vi "colourByStage.vi"(8 "error in (no error)":errorcluster, 11 "ScriptEditorV2 in":refnum<class "ScriptEditorV2.lvclass">) -> (0 "error out":errorcluster, 3 "ScriptEditorV2 out":refnum<class "ScriptEditorV2.lvclass">)   [LabVIEW 2009, in "Views.lvlib" / "ScriptEditor.lvlib" / "ScriptEditorV2.lvclass"]
uses:
  ScriptEditorV2.lvclass
  ScriptEditorV2.lvclass/ScriptEditorV2.ctl
  Tools/DatabaseHelpers/DbConnection/DeviceDataBase/deviceDataBase.lvclass
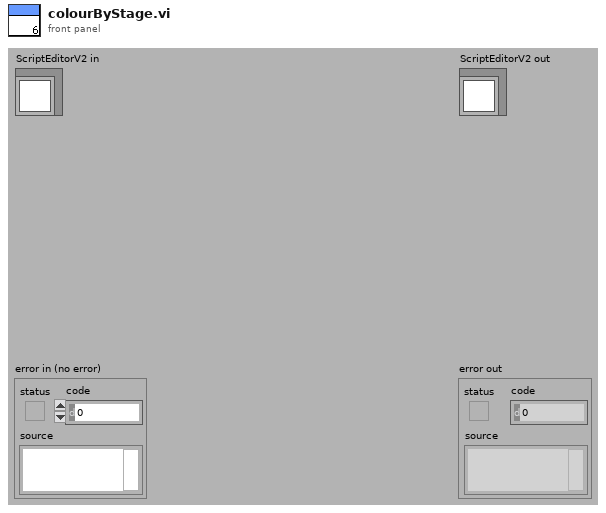
[diagram p1: front panel]
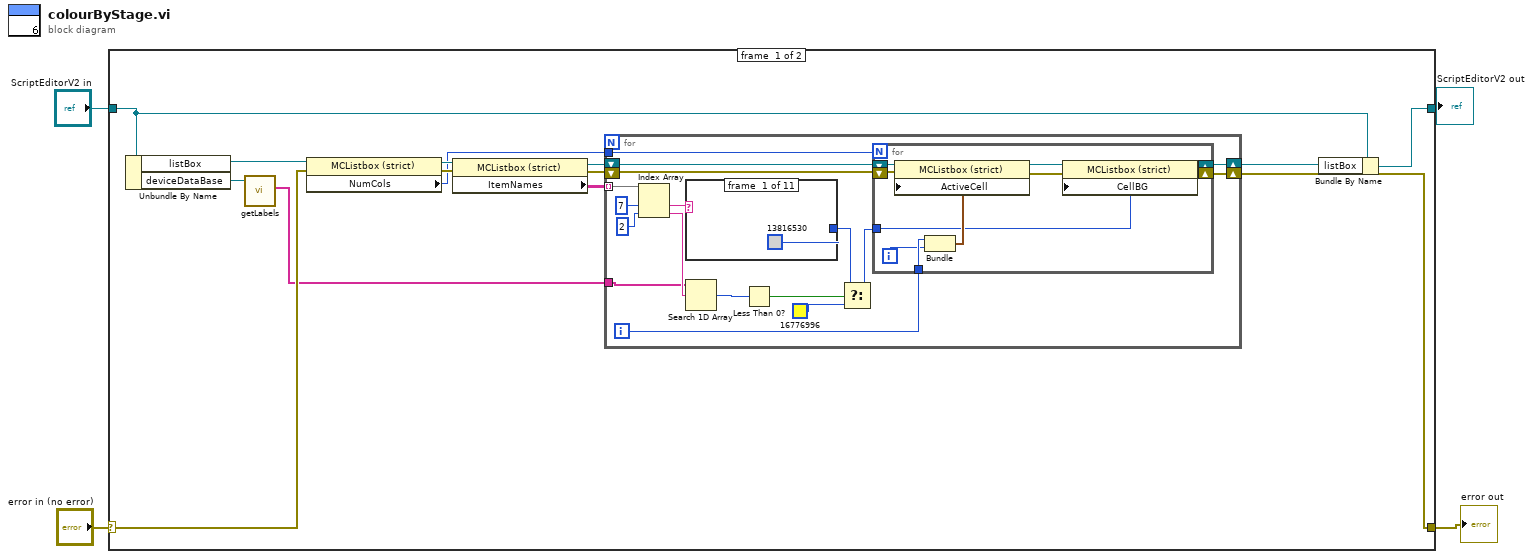
[diagram p0: block diagram]
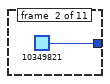
[diagram p2: hidden frame]
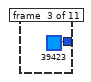
[diagram p3: hidden frame]
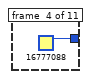
[diagram p4: hidden frame]
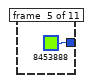
[diagram p5: hidden frame]
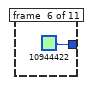
[diagram p6: hidden frame]
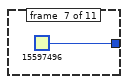
[diagram p7: hidden frame]
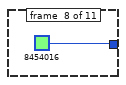
[diagram p8: hidden frame]
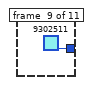
[diagram p9: hidden frame]
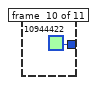
[diagram p10: hidden frame]
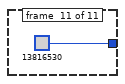
[diagram p11: hidden frame]
diagram:
  n1 = case shown="No Error" "error in (no error)" {
    selector: "error in (no error)" -> [w14 w58]
    tunnel: [w7 w58] -> w3
    tunnel: [w10 w57] -> w1
    tunnel: "ScriptEditorV2 in" -> [w11 w57]
    frame #0 {
      n2 = Unbundle By Name(w11) -> ("listBox"=w13:refnum<vi>, "deviceDataBase"=w6:refnum<class "deviceDataBase.lvclass">)
      n3 = call "getLabels.vi"("deviceDataBase in"=w6) -> ("labels"=w5:string[])  [unwired: 8 in, 2 out]
      n4 = property class="MCListbox (strict)"(reference=w13, error in=w14) -> (reference out=w16:refnum<vi>, error out=w15:errorcluster, "NumCols"=w12:u32)
      n5 = property class="MCListbox (strict)"(reference=w16, error in=w15) -> (reference out=w17:refnum<vi>, error out=w8:errorcluster, "ItemNames"=w18:string[][])
      n6 = for {
        tunnel: w18 -> [w35] mode=indexing
        tunnel: w12 -> [w31]
        shift-right: [w29] -> w9
        shift-left: w17 -> [w32]
        shift-right: [w27] -> w7
        shift-left: w8 -> [w28]
        tunnel: w5 -> [w24]
        i -> [w30]
        n7 = Index Array(array=w35, index #1=7, index #2=2) -> (element #1=w33:string, element #2=w25:string)
        n8 = case shown="\"Manipulation\"" w33 {
          tunnel: [u32 13816530 u32 10349821 u32 39423 u32 16777088 u32 8453888 u32 10944422 u32 15597496 u32 8454016 u32 9302511 u32 10944422 u32 13816530] -> w21
          frame #0 {
          }
          frame #1 {
          }
          frame #2 {
          }
          frame #3 {
          }
          frame #4 {
          }
          frame #5 {
          }
          frame #6 {
          }
          frame #7 {
          }
          frame #8 {
          }
          frame #9 {
          }
          frame #10 {
          }
        }
        n9 = Search 1D Array(1D array=w24, element=w25) -> (index of element=w22:i32)  [unwired: 1 in]
        n10 = Less Than 0?(x=w22) -> (x < 0?=w23:bool)
        n11 = Select(t=w21, s=w23, f=u32 16776996) -> (s? t:f=w20:u32)
        n12 = for {
          N: w31 -> [_]
          tunnel: w30 -> [w37]
          shift-right: [w41] -> w29
          shift-left: w32 -> [w44]
          shift-right: [w39] -> w27
          shift-left: w28 -> [w40]
          tunnel: w20 -> [w38]
          i -> [w36]
          n13 = Bundle(w37, w36) -> (w42:cluster{i32, i32})  [unwired: 1 in]
          n14 = property class="MCListbox (strict)"(reference=w44, error in=w40, "ActiveCell"=w42) -> (reference out=w45:refnum<vi>, error out=w43:errorcluster)
          n15 = property class="MCListbox (strict)"(reference=w45, error in=w43, "CellBG"=w38) -> (reference out=w41:refnum<vi>, error out=w39:errorcluster)
        }
      }
      n16 = Bundle By Name(cluster=w11, "listBox"=w9) -> (w10:refnum<class "ScriptEditorV2.lvclass">)
    }
    frame #1 {
    }
  }
  "error out" <- w3
  "ScriptEditorV2 out" <- w1
